vi "New Path Ubication.vi"() -> (2 "path string":string, 3 "path":path)   [LabVIEW 2020, in "Control de MaP.lvlib"]
uses:
  Control de MaP.lvlib
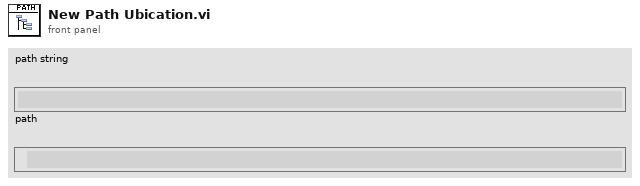
[diagram p1: front panel]
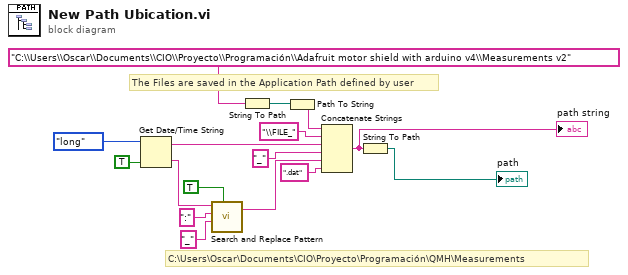
[diagram p0: block diagram]
diagram:
  # "C:\\Users\\Oscar\\Documents\\CIO\\Proyecto\\Programación\\QMH\\Measurements"
  # "The Files are saved in the Application Path defined by user"
  n1 = Get Date/Time String(date format (0)=enum16{"short", "long", "abbreviated"}."long", want seconds? (F)=TRUE) -> (date string=w8:string, time string=w11:string)  [unwired: 1 in]
  n2 = call <vilib>:"Search and Replace Pattern.vi"("string"=w11, "regular expression (\"\")"=":" ("regular expression (\"\")"), "replace string (\"\")"="_" ("replace string (\"\")"), "replace all? (F)"=TRUE) -> ("result string"=w14:string)  [unwired: 1 in, 1 out]
  n3 = String To Path(string="C:\\Users\\Oscar\\Documents\\CIO\\Proyecto\\Programación\\Adafruit motor shield with arduino v4\\Measurements v2") -> (path=w1:path)
  n4 = Path To String(path=w1) -> (string=w6:string)
  n5 = Concatenate Strings(w6, "\\FILE_" ("string"), w8, "_" ("string"), w14, ".dat" ("string")) -> (w16:string)
  "path string" <- w16
  n6 = String To Path(string=w16) -> (path=→"path":path)
